vi "peaks batch.vi"(0 "signal in":dbl[](array[numeric]) format="%.2f", 5 "Min Peak Area":dbl min=0.0 format="%.2f", 7 "X Interval":dbl=1.0 format="%.4f", 9 "tuning parameters":T3 {"peak threshold" min=0.0 format="%.2f"; "max noise" min=0.0 format="%.2f"}) -> (4 "signal out":dbl[](array[numeric]) format="%.2f", 10 "Peaks":T2(array[cluster]) {"Area" format="%.4f"; "Summit Y" format="%.4f"; "End Y" format="%.4f"; "End X" format="%.4f"; "Summit X" format="%.4f"; "Start Y" format="%.4f"; "Start X" format="%.4f"}, 15 "graph data":cluster{cluster{"X":dbl, "Y":dbl}[]}[](array[cluster]) {"?"."X" format="%.4f"; "?"."Y" format="%.2f"})   [LabVIEW 2012]
uses:
  Tuning.ctl
panel:
  in  "?":T1 {"Area" format="%.4f"; "Summit Y" format="%.4f"; "End Y" format="%.4f"; "End X" format="%.4f"; "Summit X" format="%.4f"; "Start Y" format="%.4f"; "Start X" format="%.4f"}
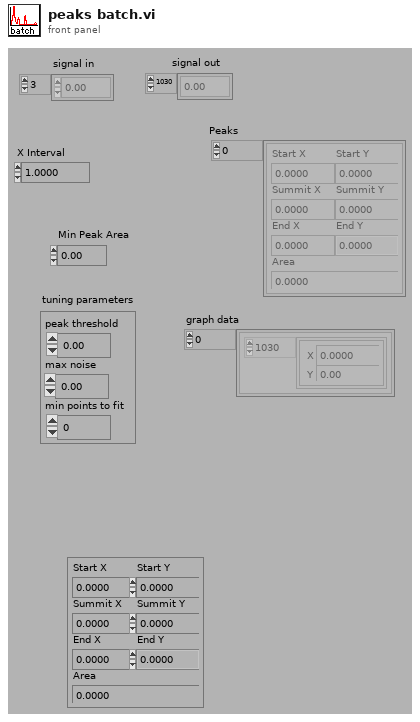
[diagram p1: front panel]
types:
  T1 = cluster{"Start X":dbl, "Start Y":dbl, "Summit X":dbl, "Summit Y":dbl, "End X":dbl, "End Y":dbl, "Area":dbl}
  T2 = cluster{"Start X":dbl, "Start Y":dbl, "Summit X":dbl, "Summit Y":dbl, "End X":dbl, "End Y":dbl, "Area":dbl}[]
  T3 = typedef "Tuning.ctl" = cluster{"max noise":dbl, "min points to fit":i32, "peak threshold":dbl}
  T4 = typedef "XY Plot.ctl" = cluster{"X":dbl, "Y":dbl}[]
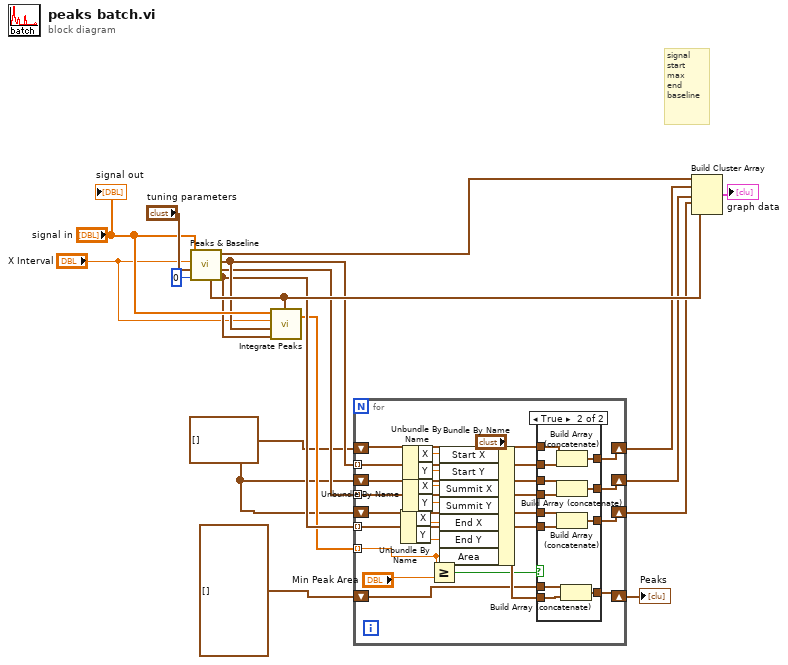
[diagram p0: block diagram]
diagram:
  w3 = cluster{"X":dbl, "Y":dbl}[] []
  # "signal\nstart\nmax\nend\nbaseline"
  n1 = call "Peaks & Baseline.vi"("Y data"="signal in", "X interval (1.0)"="X Interval", "tuning parameters\n(0:auto-calc)"="tuning parameters", "iteration (0:init)"=0) -> ("baseline"=w13:T4, "X,Y data"=w14:T4, "peak starts"=w11:T4, "peak maxima"=w10:T4, "peak ends"=w9:T4)  [unwired: 2 in]
  n2 = call "Integrate Peaks.vi"("Y data"="signal in", "X interval"="X Interval", "peak starts"=w11, "peak ends"=w9, "baseline"=w13) -> ("peak areas"=w8:dbl[])  [unwired: 1 in]
  n3 = for {
    tunnel: w11 -> [w24] mode=indexing
    tunnel: w10 -> [w25] mode=indexing
    tunnel: w9 -> [w26] mode=indexing
    tunnel: w8 -> [w31] mode=indexing
    shift-right: [w27] -> w7
    shift-left: T2 [] -> [w28]
    shift-right: [w18] -> w6
    shift-left: w3 -> [w23]
    shift-right: [w19] -> w5
    shift-left: w3 -> [w22]
    shift-right: [w20] -> w4
    shift-left: w3 -> [w21]
    n4 = Unbundle By Name(w26) -> ("X"=w33:dbl, "Y"=w32:dbl)
    n5 = Unbundle By Name(w24) -> ("X"=w37:dbl, "Y"=w36:dbl)
    n6 = Unbundle By Name(w25) -> ("X"=w35:dbl, "Y"=w34:dbl)
    n7 = Greater Or Equal?(x=w31, y="Min Peak Area") -> (x >= y?=w29:bool)
    n8 = Bundle By Name(cluster="?", "Start X"=w37, "Start Y"=w36, "Summit X"=w35, "Summit Y"=w34, "End X"=w33, "End Y"=w32, "Area"=w31) -> (w38:T1)
    n9 = case shown="True" w29 {
      tunnel: w38 -> [_ w55]
      tunnel: w28 -> [w43 w54]
      tunnel: [w43 w53] -> w27
      tunnel: w26 -> [_ w52]
      tunnel: w25 -> [_ w51]
      tunnel: w24 -> [_ w50]
      tunnel: w23 -> [w42 w49]
      tunnel: w22 -> [w41 w48]
      tunnel: w21 -> [w40 w47]
      tunnel: [w40 w46] -> w20
      tunnel: [w41 w45] -> w19
      tunnel: [w42 w44] -> w18
      frame False {
      }
      frame True {
        n10 = Build Array (concatenate)(w49, w50) -> (w44:cluster{"X":dbl, "Y":dbl}[])
        n11 = Build Array (concatenate)(w48, w51) -> (w45:cluster{"X":dbl, "Y":dbl}[])
        n12 = Build Array (concatenate)(w47, w52) -> (w46:cluster{"X":dbl, "Y":dbl}[])
        n13 = Build Array (concatenate)(w54, w55) -> (w53:T2)
      }
    }
  }
  "Peaks" <- w7
  n14 = Build Cluster Array(w14, w6, w5, w4, w13) -> (→"graph data":cluster{"baseline":T4}[])
  "signal out" <- "signal in"
